vi "Get DC Pins.vi"(8 "error in (no error)":errorcluster, 11 "QPA Measurement in":refnum<class "QPA Measurement.lvclass">) -> (0 "error out":errorcluster, 3 "QPA Measurement out":refnum<class "QPA Measurement.lvclass">)   [LabVIEW 2016, in "QPA Measurement.lvlib" / "QPA Measurement.lvclass"]
uses:
  QPA Measurement.lvclass
  C:/Projects/STS/Common/Sequence Automation/Plugins/Measurement Interface.lvlibp/Measurement Interface.lvclass
  QPA Measurement.lvclass/QPA Measurement.ctl
  Plugins/Measurement Interface.lvlibp/Private Methods/Active Sequence File/Read Active Sequence File.vi
  Plugins/TestStand API Tools (TSAT).lvlibp/Sequence File Actions/TSAT Sequence File Actions.lvlib
  Plugins/TestStand API Tools (TSAT).lvlibp/TSAT Utilities/TSAT Utilities.lvlib
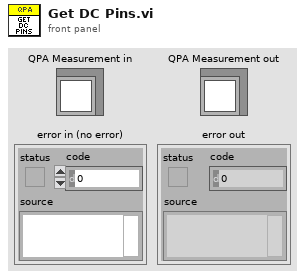
[diagram p1: front panel]
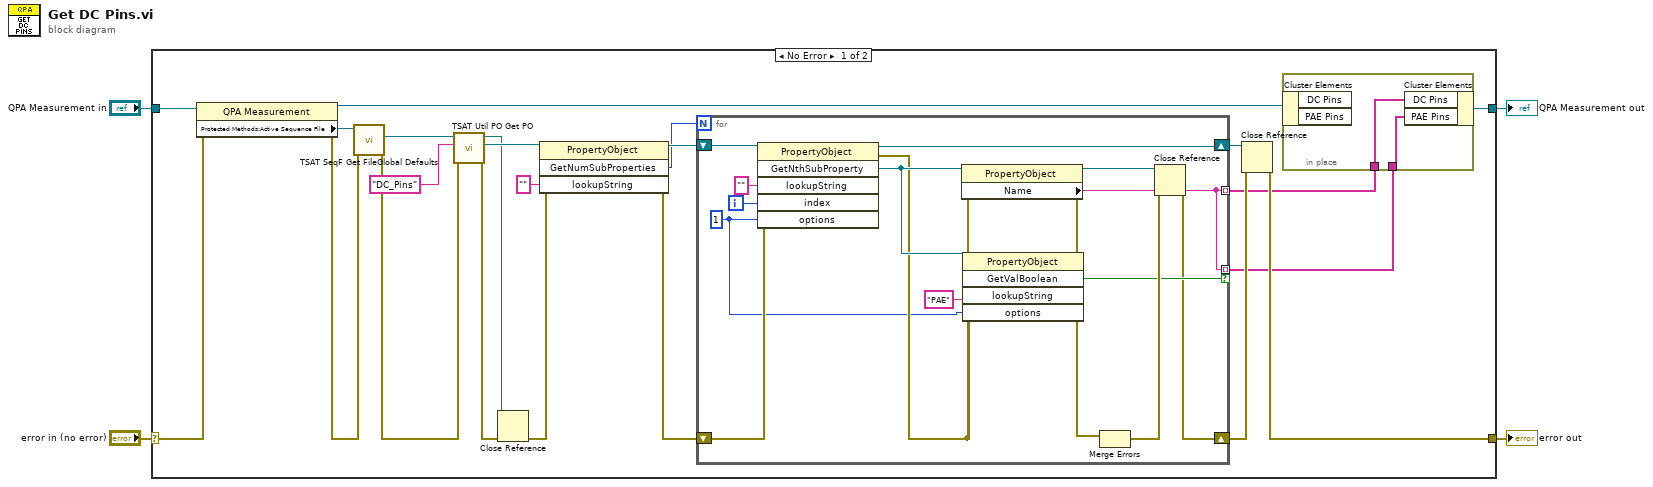
[diagram p0: block diagram]
diagram:
  n1 = case shown="No Error" "error in (no error)" {
    selector: "error in (no error)" -> [w25 w46]
    tunnel: [w15 w46] -> w3
    tunnel: [w10 w45] -> w1
    tunnel: "QPA Measurement in" -> [w26 w45]
    frame No Error {
      n2 = property class="QPA Measurement"(reference=w26, error in=w25) -> (reference out=w11:refnum<class "QPA Measurement.lvclass">, error out=w23:errorcluster, "Protected Methods:Active Sequence File"=w24:refnum<k7>)
      n3 = call "TSAT SeqF Get FileGlobal Defaults.vi"("Error In"=w23, "Sequence File In"=w24) -> ("Error Out"=w20:errorcluster, "FileGlobalsDefaultValues"=w22:refnum<k7>)  [unwired: 7 in, 1 out]
      n4 = call "TSAT Util PO Get PO.vi"("error in (no error)"=w20, "Sub Property to Retrieve"="DC_Pins", "Property Object in"=w22) -> ("error out"=w13:errorcluster, "SubProperty"=w19:refnum<k7>, "PropertyObjectOut"=w5:refnum<k7>)  [unwired: 6 in]
      n5 = Close Reference(reference=w5, error in (no error)=w13) -> (error out=w6:errorcluster)
      n6 = invoke class="PropertyObject" method="GetNumSubProperties"(reference=w19, error in=w6, "lookupString"="") -> (reference out=w18:refnum<k7>, error out=w12:errorcluster, "GetNumSubProperties"=w14:i32)  [unwired: 1 in, 1 out]
      n7 = for {
        N: w14 -> [_]
        shift-right: [w41] -> w17
        shift-left: w18 -> [w44]
        shift-right: [w33] -> w16
        shift-left: w12 -> [w40]
        tunnel: [w34] -> w8 mode=indexing if=w35
        tunnel: [w34] -> w9 mode=indexing
        i -> [w30]
        w29 = 1 ("options")
        n8 = invoke class="PropertyObject" method="GetNthSubProperty"(reference=w44, error in=w40, "lookupString"="", "index"=w30, "options"=w29) -> (reference out=w41:refnum<k7>, error out=w39:errorcluster, "GetNthSubProperty"=w43:refnum<k7>)  [unwired: 1 in, 3 out]
        n9 = property class="PropertyObject"(reference=w43, error in=w39) -> (reference out=w32:refnum<k7>, error out=w38:errorcluster, "Name"=w34:string)
        n10 = invoke class="PropertyObject" method="GetValBoolean"(reference=w43, error in=w39, "lookupString"="PAE", "options"=w29) -> (error out=w37:errorcluster, "GetValBoolean"=w35:bool)  [unwired: 1 in, 3 out]
        n11 = Merge Errors(w38, w37) -> (w36:errorcluster)
        n12 = Close Reference(reference=w32, error in (no error)=w36) -> (error out=w33:errorcluster)
      }
      n13 = Close Reference(reference=w17, error in (no error)=w16) -> (error out=w15:errorcluster)
      n14 = in-place {
        in-place-border: w9 -> [w28]
        in-place-border: w8 -> [w27]
        n15 = in-place-cluster #1(w11) -> ()  [unwired: 2 out]
        n16 = in-place-cluster #1("DC Pins"=w28, "PAE Pins"=w27) -> (w10:refnum<class "QPA Measurement.lvclass">)
      }
    }
    frame Error {
    }
  }
  "error out" <- w3
  "QPA Measurement out" <- w1
